vi "visionScrew.vi"(3 "Error In":errorcluster, 4 "Aim_Color":string="Default") -> (0 "Error Out":errorcluster, 2 "Position":string)   [LabVIEW 2019]
uses:
  WSCbot_V3_Toolkit.lvlibp
panel:
  out "Classes (Color Classification 1)":string[](array[string])
  out "Finish?":bool
  out "original":T1(plugin-control)
  out "target position":i32
  out "Image Out":T1(plugin-control)
  in  "Stop (F)":bool
  # "0        1\n\n2        3"
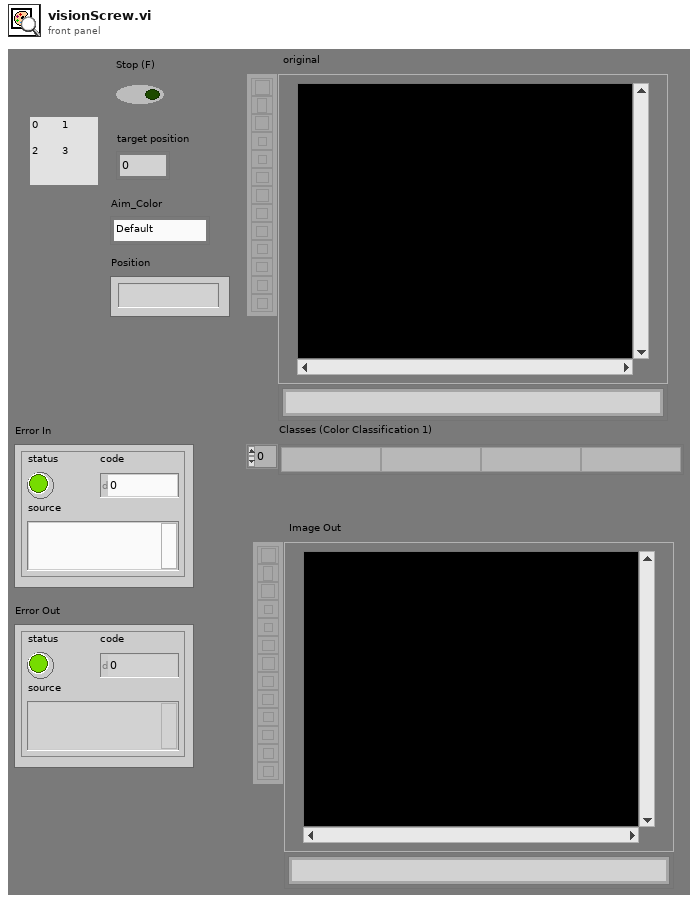
[diagram p1: front panel]
types:
  T1 = typedef "IMAQ Image.ctl" = refnum<image>
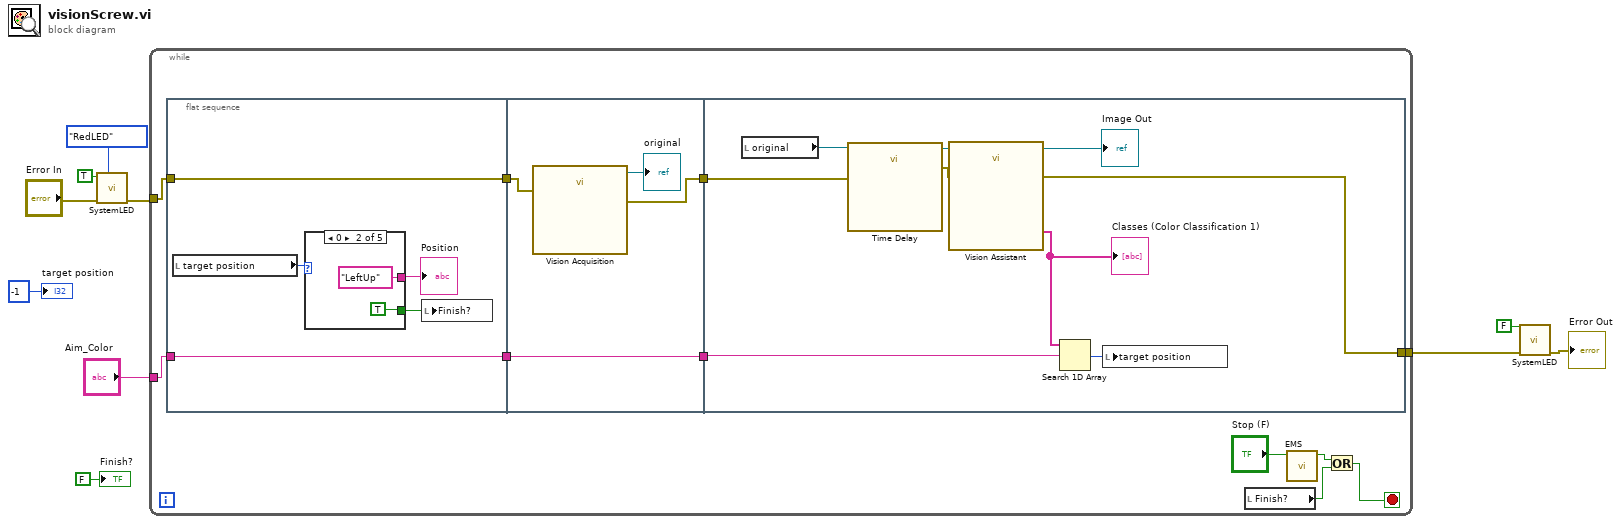
[diagram p0: block diagram]
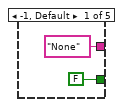
[diagram p2: hidden frame]
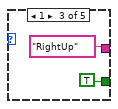
[diagram p3: hidden frame]
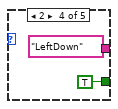
[diagram p4: hidden frame]
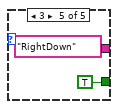
[diagram p5: hidden frame]
diagram:
  n1 = call "SystemLED.vi"("SelectColor"=enum16{"RedLED", "GreenLED", "YellowLED"}."RedLED", "error in"="Error In", "Set"=TRUE) -> ("error out"=w2:errorcluster)  [unwired: 8 in]
  n2 = while {
    tunnel: w2 -> [w20]
    tunnel: "Aim_Color" -> [w21]
    tunnel: [w11] -> w1
    stop <- w12 stop-if-true
    n3 = flat-sequence {
      tunnel: w20 -> [w25]
      tunnel: w21 -> [w26]
      tunnel: [w26] -> w19
      tunnel: [w25] -> w17
      tunnel: w19 -> [w40]
      tunnel: [w40] -> w18
      tunnel: w17 -> [w38]
      tunnel: [w37] -> w16
      tunnel: w18 -> [w48]
      tunnel: w16 -> [w44]
      tunnel: [w41] -> w11
      frame #0 {
        n4 = local read "target position"() -> (w24:i32)
        n5 = case shown="0" w24 {
          tunnel: ["None" "LeftUp" "RightUp" "LeftDown" "RightDown"] -> w23
          tunnel: [FALSE TRUE TRUE TRUE TRUE] -> w22
          frame -1, Default {
          }
          frame 0 {
          }
          frame 1 {
          }
          frame 2 {
          }
          frame 3 {
          }
        }
        "Position" <- w23
        n6 = local write "Finish?"(w22) -> ()
      }
      frame #1 {
        n7 = call "Vision Acquisition"("error in"=w38) -> ("Image Out"=→"original":T1, "error out"=w37:errorcluster)  [unwired: 25 in]
      }
      frame #2 {
        n8 = local read "original"() -> (w43:T1)
        n9 = call "Time Delay"("error in (no error)"=w44) -> ("error out"=w42:errorcluster)  [unwired: 10 in]
        n10 = call "Vision Assistant"("Image In"=w43, "error in"=w42) -> ("Image Out"=→"Image Out":T1, "Classes (Color Classification 1)"=w45:string[], "error out"=w41:errorcluster)  [unwired: 23 in]
        "Classes (Color Classification 1)" <- w45
        n11 = Search 1D Array(1D array=w45, element=w48) -> (index of element=w46:i32)  [unwired: 1 in]
        n12 = local write "target position"(w46) -> ()
      }
    }
    n13 = local read "Finish?"() -> (w15:bool)
    n14 = call "EMS.vi"("ProgramStop"="Stop (F)") -> ("EMS"=w13:bool)  [unwired: 9 in, 1 out]
    n15 = Or(x=w13, y=w15) -> (x .or. y?=w12:bool)
  }
  n16 = call "SystemLED.vi"("error in"=w1, "Set"=FALSE) -> ("error out"=→"Error Out":errorcluster)  [unwired: 9 in]
  "Finish?" <- FALSE ("Finish?")
  "target position" <- -1 ("target position")
